vi "nelder_evaluate_point.vi"(8 "error in":errorcluster, 9 "settling time":u32, 10 "point":sgl[][](array[numeric]), 11 "refs":T2) -> (0 "error out":errorcluster, 3 "f_Val":dbl)   [LabVIEW 2018]
uses:
  C:/Program Files/National Instruments/LabVIEW 2018/instr.lib/IDS/ueye.NET/uEyeDotNet.dll
  <userlib>/PDamp/PDref.ctl
  <userlib>/PDamp/channel.ctl
panel:
  out "ypos":sgl
  out "zpos":sgl
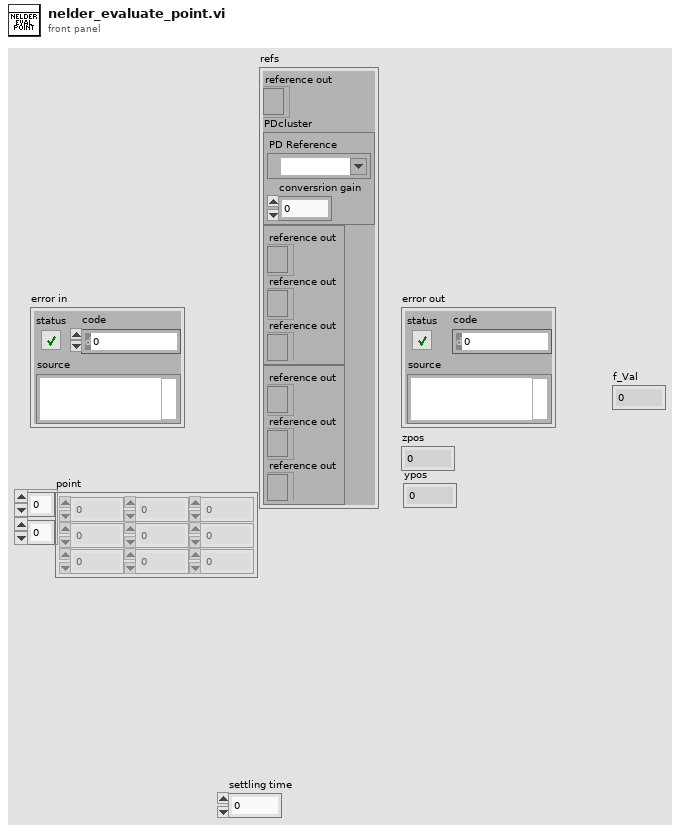
[diagram p1: front panel]
types:
  T1 = typedef "PDref.ctl" = cluster{"PD Reference":refnum<visa-resource-name>, "conversrion gain":dbl}
  T2 = cluster{"reference out":refnum<k24>, "PDcluster":T1, cluster{"reference out":refnum<k7>, "reference out":refnum<k7>, "reference out":refnum<k7>}, cluster{"reference out":refnum<k7>, "reference out":refnum<k7>, "reference out":refnum<k7>}}
  T3 = cluster{"reference out":refnum<k7>, "reference out":refnum<k7>, "reference out":refnum<k7>}
  T4 = typedef "channel.ctl" = enum16{"ch1", "ch2", "ch3", "ch4"}
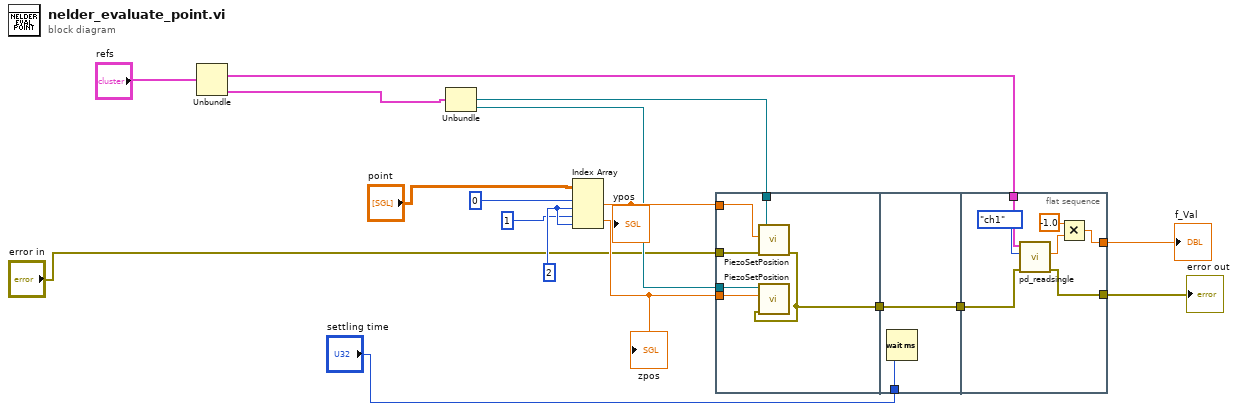
[diagram p0: block diagram]
diagram:
  w16 = 2 ("disabled index (col)")
  n1 = Unbundle("refs") -> ("PDcluster"=w7:T1, w8:T3)  [unwired: 2 out]
  n2 = Unbundle(w8) -> ("reference out"=w11:refnum<k7>, "reference out"=w10:refnum<k7>)  [unwired: 1 out]
  n3 = Index Array(array="point", index (row) #1=0 ("disabled index (row)"), index (col) #1=w16, index (row) #2=1 ("disabled index (row)"), index (col) #2=w16) -> (element #1=w13:sgl, element #2=w12:sgl)
  "zpos" <- w12
  "ypos" <- w13
  n4 = flat-sequence {
    tunnel: w13 -> [w23]
    tunnel: w12 -> [w22]
    tunnel: w11 -> [w21]
    tunnel: w10 -> [w20]
    tunnel: [w19] -> w4
    tunnel: "error in" -> [w18]
    tunnel: "settling time" -> [w25]
    tunnel: [w24] -> w5
    tunnel: w4 -> [w24]
    tunnel: w7 -> [w32]
    tunnel: [w26] -> w6
    tunnel: w5 -> [w30]
    tunnel: [w29] -> w2
    frame #0 {
      n5 = call <userlib>:"PiezoSetPosition.vi"("error in (no error)"=w18, "pos in"=w23, "reference"=w21) -> ("error out"=w19:errorcluster)  [unwired: 3 in, 1 out]
      n6 = call <userlib>:"PiezoSetPosition.vi"("error in (no error)"=w19, "pos in"=w22, "reference"=w20) -> ()  [unwired: 3 in, 2 out]
    }
    frame #1 {
      n7 = Wait (ms)(milliseconds to wait=w25) -> ()  [unwired: 1 out]
    }
    frame #2 {
      n8 = call <userlib>:"pd_readsingle.vi"("PDcluster in"=w32, "channel"=channel."ch1", "error in (no error)"=w30) -> ("photocurrent"=w28:dbl, "error out"=w29:errorcluster)  [unwired: 5 in, 1 out]
      n9 = Multiply(x=-1.0, y=w28) -> (x*y=w26:dbl)
    }
  }
  "f_Val" <- w6
  "error out" <- w2
